vi "To String Array.vi"(8 "error in (no error)":errorcluster, 11 "Parallel Step Config in":refnum<class "Parallel Step Config.lvclass">) -> (0 "error out":errorcluster, 1 "Step String Array":string[](array[string]), 3 "Parallel Step Config out":refnum<class "Parallel Step Config.lvclass">)   [LabVIEW 2015, in "Parallel Step Config.lvclass"]
uses:
  Parallel Step Config.lvclass
  classes/Step/Config/Step Config.lvclass
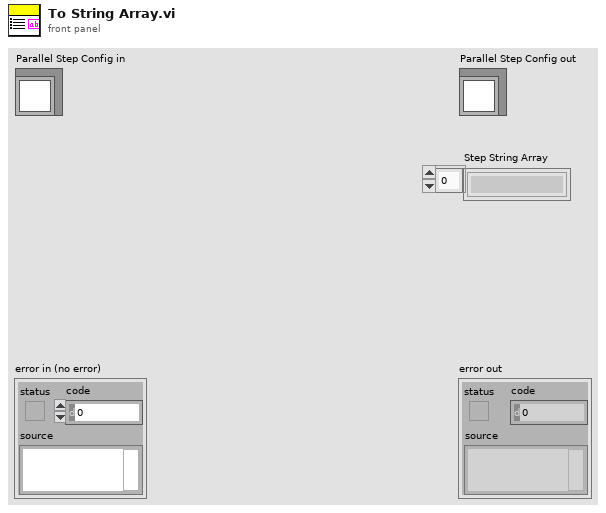
[diagram p1: front panel]
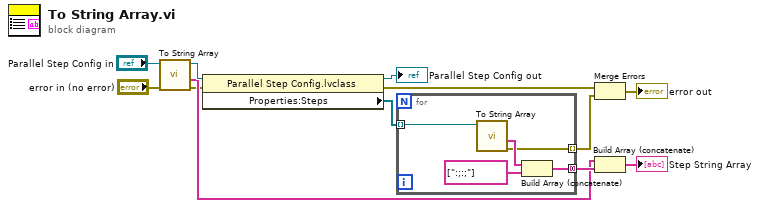
[diagram p0: block diagram]
diagram:
  n1 = call-parent "To String Array.vi"("error in (no error)"="error in (no error)", "Step Config in"="Parallel Step Config in") -> ("error out"=w1:errorcluster, "Step String Array"=w6:string[], "Step Config out"=w10:refnum<class "Parallel Step Config.lvclass">)  [unwired: 7 in]
  n2 = property class="Parallel Step Config.lvclass"(reference=w10, error in=w1) -> (reference out=→"Parallel Step Config out":refnum<class "Parallel Step Config.lvclass">, error out=w2:errorcluster, "Properties:Steps"=w8:refnum<class "Step Config.lvclass">[])
  n3 = for {
    tunnel: w8 -> [w17] mode=indexing
    tunnel: [w14] -> w7 mode=concatenating
    tunnel: [w13] -> w4 mode=indexing
    n4 = call-dynamic "To String Array.vi"("Step Config in"=w17) -> ("error out"=w13:errorcluster, "Step String Array"=w16:string[])  [unwired: 8 in, 1 out]
    n5 = Build Array (concatenate)(w16, string[] [":;:;"] ("array")) -> (w14:string[])
  }
  n6 = Merge Errors(w2, w4) -> (→"error out":errorcluster)
  n7 = Build Array (concatenate)(w6, w7) -> (→"Step String Array":string[])
